vi "Process waveform API.vi"(8 "Error In":errorcluster, 11 "Waveform + name 2":T1) -> (0 "Error Out":errorcluster)   [LabVIEW 2017, in "Processing.lvlib"]
uses:
  Processing.lvlib
  Controls/Command Data [cluster].ctl
  Controls/Commands [enum].ctl
  Events/Events.lvlib
panel:
  in  "Waveform + name":T2
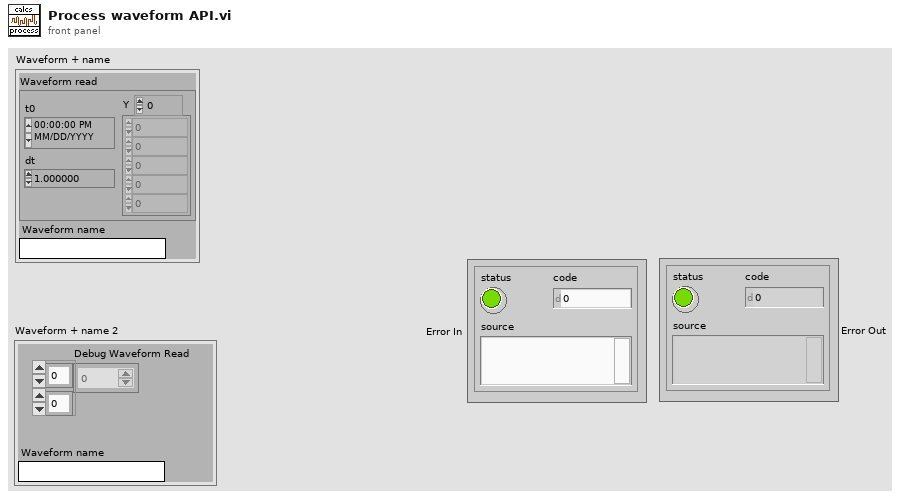
[diagram p1: front panel]
types:
  T1 = cluster{"Debug Waveform Read":dbl[][], "Waveform name":string}
  T2 = cluster{"Waveform read":waveform(dbl), "Waveform name":string}
  T3 = typedef "Processing.lvlib/Command Data [cluster].ctl" = cluster{"Command":T4, "Data":variant}
  T4 = typedef "Processing.lvlib/Commands [enum].ctl" = enum16{"Start", "Stop", "Process waveform", "Scope A-B processing", "DAQ A-B processing", "DAQ-Scope Stitching", "Update Test Info"}
  T5 = typedef "Events.lvlib/Refs [cluster].ctl" = cluster{"Exit":refnum<user-event>, "Controller":refnum<user-event>, "System Error":refnum<user-event>, "UI":refnum<user-event>, "Example Module":refnum<user-event>, "Shutter":refnum<user-event>, "Monochromator":refnum<user-event>, "DAQ":refnum<user-event>, "Scope":refnum<user-event>, "Processing":refnum<user-event>, "File IO":refnum<user-event>, "Colour wheel":refnum<user-event>}
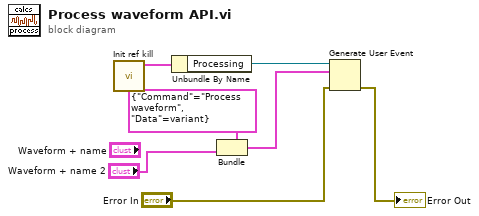
[diagram p0: block diagram]
diagram:
  n1 = call "Init ref kill.vi"() -> ("Messages"=w7:T5)  [unwired: 10 in, 1 out]
  n2 = Unbundle By Name(w7) -> ("Processing"=w6:refnum<user-event>)
  n3 = Bundle(cluster=T3 {"Command"=enum."Process waveform", "Data"=variant} ("event data"), "Data"="Waveform + name 2") -> (w4:T3)  [unwired: 1 in]
  n4 = Generate User Event(user event=w6, event data cluster=w4, error in="Error In") -> (error out=→"Error Out":errorcluster)  [unwired: 1 in, 1 out]
